vi "Get PString.vi"(9 "offset (0)":i32, 11 "bytes":refnum<class "Bytes.lvclass">) -> (1 "offset past PString":i32, 2 "PString":string, 3 "Bytes out":refnum<class "Bytes.lvclass">)   [LabVIEW 2020, in "lvdata.lvlib"]
doc: "Returns the PString starting at offset."
uses:
  lvdata.lvlib
  Bytes/Bytes.lvclass
  Bytes/Bytes.lvclass/Bytes.ctl
  Bytes/from_byte_array.vi
panel:
  # "[OpenG VI Tags] ***Do Not Remove***"
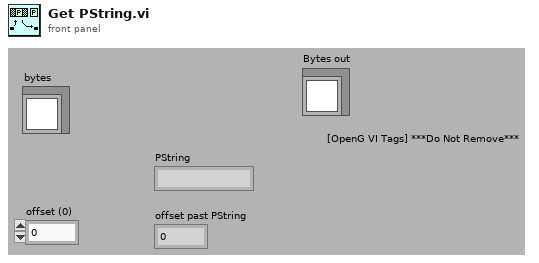
[diagram p1: front panel]
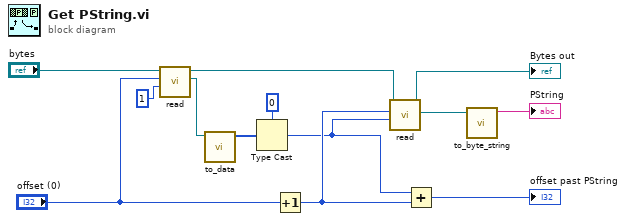
[diagram p0: block diagram]
diagram:
  n1 = call "read.vi"("length (-1: rest)"=1, "offset (-1: current position)"="offset (0)", "Bytes in"="bytes") -> ("Bytes read"=w10:refnum<class "Bytes.lvclass">, "Bytes out"=w1:refnum<class "Bytes.lvclass">)  [unwired: 7 in]
  n2 = call "to_data.vi"("Bytes in"=w10) -> ("byte array"=w9:u8[])  [unwired: 10 in]
  n3 = Type Cast(type=u8 0 ("element"), x=w9) -> (*(type *) &x=w4:u8)
  n4 = Increment(x="offset (0)") -> (x+1=w7:i32)
  n5 = call "read.vi"("length (-1: rest)"=w4, "offset (-1: current position)"=w7, "Bytes in"=w1) -> ("Bytes read"=w6:refnum<class "Bytes.lvclass">, "Bytes out"=→"Bytes out":refnum<class "Bytes.lvclass">)  [unwired: 7 in]
  n6 = Add(x=w4, y=w7) -> (x+y=→"offset past PString":i32)
  n7 = call "to_byte_string.vi"("Bytes in"=w6) -> ("byte string"=→"PString":string)  [unwired: 10 in]
